vi "fake tool ignored.vi"() -> ()   [LabVIEW 2025, in "MCP Server tests.lvlib"]
doc: "this is a tool ignoring some in- and outputs. If you see Input1 and Output1, the ignoring didnt work."
uses:
  MCP Server tests.lvlib
panel:
  out "Output1":string
  in  "Input1":string
  out "output string":string
  in  "input string":string
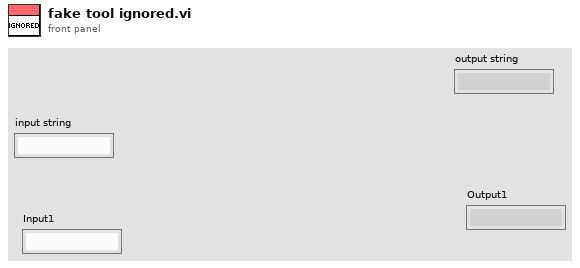
[diagram p1: front panel]
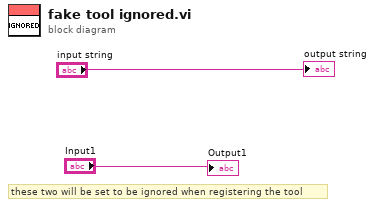
[diagram p0: block diagram]
diagram:
  # "these two will be set to be ignored when registering the tool"
  "output string" <- "input string"
  "Output1" <- "Input1"
